vi "toXML.vi"(8 "error in (no error)":errorcluster, 11 "Point in":refnum<class "Point.lvclass">) -> (0 "error out":errorcluster, 2 "xmlNode":refnum<class "xmlNode.lvclass">, 3 "Point out":refnum<class "Point.lvclass">)   [LabVIEW 2011, in "Tools.lvlib" / "Sequencing.lvlib" / "Point.lvclass"]
uses:
  Point.lvclass
  xmlNode/xmlNode.lvclass
  Point.lvclass/Point.ctl
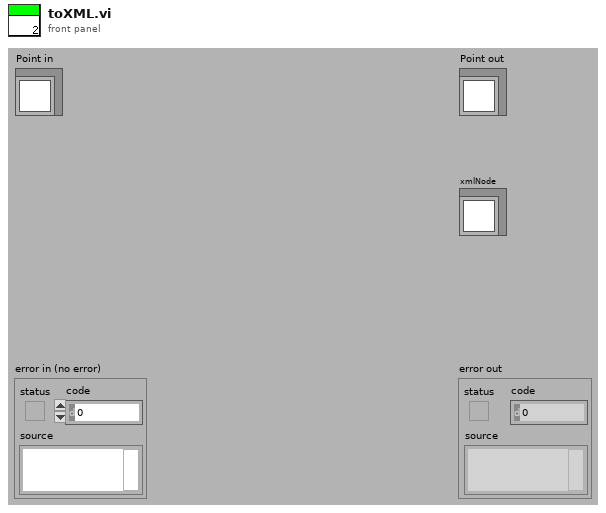
[diagram p1: front panel]
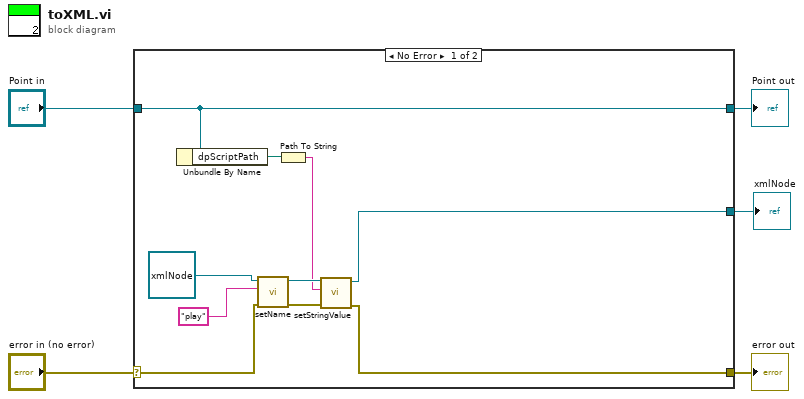
[diagram p0: block diagram]
diagram:
  n1 = case shown="No Error" "error in (no error)" {
    selector: "error in (no error)" -> [w12 w17]
    tunnel: [w7 w17] -> w4
    tunnel: [w11 w16] -> w2
    tunnel: "Point in" -> [w11 w16]
    tunnel: [w6 _] -> w1
    frame No Error {
      n2 = Unbundle By Name(w11) -> ("dpScriptPath"=w10:path)
      n3 = call-dynamic "setName.vi"("error in (no error)"=w12, "name"="play", "xmlNode.lvclass in"=refnum<class "xmlNode.lvclass"> refnum ("Tools.lvlib:xml.lvlib:xmlNode.lvclass")) -> ("error out"=w13:errorcluster, "xmlNode.lvclass out"=w14:refnum<class "xmlNode.lvclass">)  [unwired: 7 in]
      n4 = Path To String(path=w10) -> (string=w9:string)
      n5 = call-dynamic "setStringValue.vi"("error in (no error)"=w13, "stringValue"=w9, "xmlNode.lvclass in"=w14) -> ("error out"=w7:errorcluster, "xmlNode.lvclass out"=w6:refnum<class "xmlNode.lvclass">)  [unwired: 7 in]
    }
    frame Error {
    }
  }
  "error out" <- w4
  "Point out" <- w2
  "xmlNode" <- w1
